vi "Valid.vi"(11 "NotifierMessenger in":refnum<class "NotifierMessenger.lvclass">) -> (2 "Valid?":bool, 3 "NotifierMessenger out":refnum<class "NotifierMessenger.lvclass">)   [LabVIEW 2011, in "Messenging.lvlib" / "NotifierMessenger.lvclass"]
uses:
  NotifierMessenger.lvclass
  NotifierMessenger.lvclass/NotifierMessenger.ctl
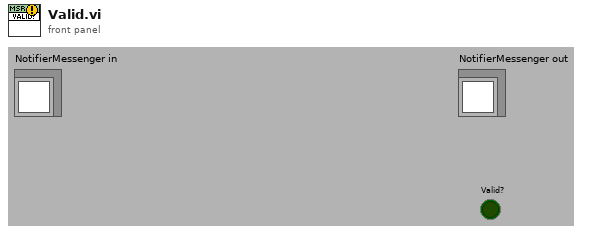
[diagram p1: front panel]
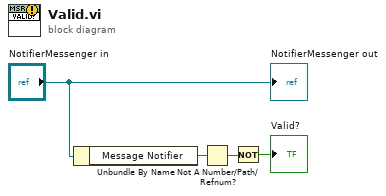
[diagram p0: block diagram]
diagram:
  n1 = Unbundle By Name("NotifierMessenger in") -> ("Message Notifier"=w4:refnum<notifier>)
  n2 = Not A Number/Path/Refnum?(number/path/refnum=w4) -> (NaN/Path/Refnum?=w3:bool)
  n3 = Not(x=w3) -> (.not. x?=→"Valid?":bool)
  "NotifierMessenger out" <- "NotifierMessenger in"
